vi "Save EPR Data-Rev3.vi"(5 "Save Data Type":T1, 7 "Spectral Data":T2={"PDT Amp [v]"=0.0, "RIS Amp [v]"=0.0, "B-Field"=[], "All In-Phase Scan Spectra"=[], "Model Select"=enum."OneCompRISTwoPDT", "Fit Each Scan"=FALSE, "PDT Center [g]"=0.0, "In-Phase Average Spectra"=[], "In-Phase Median Spectra"=[], "Out-Phase Median Spectra"=[], "Out-Phase Average Spectra"=[], "Fit Spectra"=[], "Fit No-Baseline Spectra"=[], "All Out-Phase Scan Spectra"=[], "Baseline Offset Correction"=FALSE, "In-Phase Offset [v]"=0.0, "Out-Phase Offset [v]"=0.0, "Ch2 Input\n(Balance)"=[], "Ch3 Input\n(Phase)"=[], "Ch4 Input\n(AFC)"=[], "Fit Pars"=[], "Fit Pars Errors"=[], "Fit Pars Labels"=[], "Raw Scan DAQ Data"=[], "Bad Scans Indicies"=[], "Good In-Phase Scan Spectra"=[], "Good Out-Phase Scan Spectra"=[], "Bad In-Phase Scan Spectra"=[], "Bad Out-Phase Scan Spectra"=[], "Number of bad scans"=0, "Fit History"=[], "PDT Amp. History/Set [v]"=[], "RIS Amp. History/Set [v]"=[], "RIS Amp. History/Scan [v]"=[], "All Shifted B-Fields"=[], "Good Shifted B-Fields"=[], "Ch5 Input\n(SpO2)"=[], "Ch6 Input\n(BPM)"=[], "Global SNR"=0.0, "Fit Error History"=[], "SNR History"=[]} {"Global SNR" min=0.0; "PDT Center [g]" min=0.0; "RIS Amp [v]" min=0.0; "PDT Amp [v]" min=0.0}, 8 "Measurement Information":T4={"Comments"="", "Directory Input"="", "Data file path"=path "C:/Data/EPR Data", "Scripting File"=path "C:/Data/Configuration Script.csv", "Save Data"=FALSE, "Tooth size (d11) [mm]"=0.0, "Tooth size (d12) [mm]"=0.0, "Tooth size (d21) [mm]"=0.0, "Tooth size (d22) [mm]"=0.0, "Dose of Tooth [Gy]"=0.0, "Safe Shutdown?"=FALSE, "Gases Available"=[], "Database Username"="", "Database Password"="", "Database Login URL"="", "Database Upload URL"="", "Database Success URL"="", "Database XML URL"="", "Database Resonator URL"="", "Session Number"=0, "Set #"=0, "Resonator Operator"="", "Session Type"="", "Tooth/Sample ID"="", "Volunteer ID"="", "Computer Operator"="", "Volunteer Type"="", "Site/Tooth Selection (T8,T9)"="", "Resonator"="", "Measurement Site"="", "Non-standard session?"=FALSE, "EPR DAQ Version"="", "Session Path"=path "C:/Data/EPR Data", "Chosen Applied State"="", "Chosen Initial State"="", "Time of Transition"="", "DAQ Mode"=enum."Engineering", "pO2/Scan [mmHg]"=[], "pO2/Set [mmHg]"=[], "Linewidth (HWHM)/Scan [Gauss]"=[], "Linewidth (HWHM)/Set [Gauss]"=[], "pO2 Conversion"="", "Dose Calibration Cluster"={"Dose Response"={"grand_mean"=0.0292016, "slope"=0.0188720543}, "Dose Correction"={"Sex"=1, "a0"=7.719669421, "a1"=-2.746550736, "a2"=-0.186490355, "a3"=0.041922063, "a4"=-0.849147359, "a5"=0.14330063, "a6"=0.019930219, "A_n"=40.0, "H_n"=10.12, "Dose Correction"=FALSE}, "Dose Reporting"={"Reporting is"=TRUE, "sd_threshold [AU]"=0.06, "sd_model [Gy]"=0.66, "dosimetric_threshold [Gy]"=2.0, "Add intrasession errors is"=FALSE, "Prior Radiation?"=FALSE}}, "OxyChip Slope"=0.0, "OxyChip Intercept"=0.0, "QA Mode"=enum."Select QA Mode", "QA Session?"=FALSE, "Sample Type"=enum."Empty Resonator", "Report pO2/Scan"=FALSE, "Skip End Session Save"=FALSE, "Number of sites"=enum."# Probes", "Recipient Name"="", "Sender Name"="", "Recipient Email"="", "Transition State History"=[], "pO2 Report Times"=[], "Temperature [C]"=0.0, "+Error pO2/Scan [mmHg]"=[], "-Error pO2/Scan [mmHg]"=[], "+Error pO2/Set [mmHg]"=[], "-Error pO2/Set [mmHg]"=[], "Oxy Phase Exclusion Tolerance [rad]"=0.0, "Oxy Center Exclusion Tolerance [%]"=0.0, "Oxy Exclude Unacceptable"=FALSE, "Oxy Unacceptable Estimate Flags"=[], "Save Session PPT"=FALSE, "Flagged Bad Sets"=[]} {"Oxy Center Exclusion Tolerance [%]" format="%#_9g"; "Oxy Phase Exclusion Tolerance [rad]" format="%#_9g"; "Temperature [C]" format="%#_9g"; "OxyChip Intercept" format="%#_9g"; "OxyChip Slope" format="%#_9g"; "Dose Calibration Cluster"."Dose Reporting"."dosimetric_threshold [Gy]" format="%#_9g"; "Dose Calibration Cluster"."Dose Reporting"."sd_model [Gy]" format="%#_9g"; "Dose Calibration Cluster"."Dose Reporting"."sd_threshold [AU]" format="%#_9g"; "Dose Calibration Cluster"."Dose Correction"."H_n" format="%#_9g"; "Dose Calibration Cluster"."Dose Correction"."A_n" format="%#_9g"; "Dose Calibration Cluster"."Dose Correction"."a6" format="%#.9g"; "Dose Calibration Cluster"."Dose Correction"."a5" format="%#.9g"; "Dose Calibration Cluster"."Dose Correction"."a4" format="%#.9g"; "Dose Calibration Cluster"."Dose Correction"."a3" format="%#.9g"; "Dose Calibration Cluster"."Dose Correction"."a2" format="%#.9g"; "Dose Calibration Cluster"."Dose Correction"."a1" format="%#.9g"; "Dose Calibration Cluster"."Dose Correction"."a0" format="%#.9g"; "Dose Calibration Cluster"."Dose Correction"."Sex" items=["Male"=1, "Female"=0]; "Dose Calibration Cluster"."Dose Response"."slope" format="%#_9g"; "Dose Calibration Cluster"."Dose Response"."grand_mean" format="%#_9g"}, 9 "Hardware Parameters":T7={"Scan Calibration [G/V]"=0.0, "Modulation Calibration [G/V]"=0.0, "Modulation Phase [deg]"=0.0, "Modulation Frequency [Hz]"=0.0, "Attenuation [dB]"=0, "Input Channel Count"=0, "Time constant"=7, "Sensitivity"=17, "Frequency Output Voltage [V]"=0.0, "Phase Output Voltage [V]"=0.0, "Lock-in Offset Compensation"=FALSE, "RF [GHz]"=0.0, "Q Start"=0.0, "Q End"=0.0, "Balance"=0.0, "Phase Error"=0.0, "AFC Error"=0.0, "AFC"=FALSE, "Magnet Rotation"=FALSE, "Balance Scaling Factor"=1.0, "Phase Error Scaling Factor"=1.0, "AFC Error Scaling Factor"=1.0, "Frequency Counter ID"="", "Sweep Waveform"=enum."Sawtooth", "Q-Factor Scale"=0.0, " Q-Data Scale"=0.0, " Q-Data Offset"=0.0, "Magnet Rotation Slope"=0.0, "Magnet Rotation Offset"=0.0, "Phase Sweep Resolution"=0.0, "Hardware Version Number"="", "Spectrometer ID Number"=0, "Spectrometer Name"="", "Lock in Saturation"=0.0, "Balance Threshold"=0.0, "Phase Error Threshold"=0.0, "AFC Error Threshold"=0.0, "Linear Actuator Length"=0.0, "Lock-in OK?"=FALSE, "Ignore Lock-in Comm. Failure"=FALSE, "Gradient Addresses"=[], "Gradient Calibrations [G/A*mm]"=[], "Gradient Power Supplies"=[], "Lock-in Address"="", "Magnet Type"=enum."RRI", "Camera Names"=[], "Sweep Limit [Gauss]"=0.0, "Modulation Limit [Gauss]"=0.0, "Balance Threshold Exceeded?"=FALSE, "Phase Threshold Exceeded?"=FALSE, "AFC Threshold Exceeded?"=FALSE, "Consecutive Re-tune attempts"=0, "Reverse Sweep Slope [sec]"=0.0, "Reverse Sweep Offset [G]"=0.0, "AFC Field Correction [V/MHz]"=0.0, "Active Gradients (X Y Z)"=[], "SpO2 Calibration [SpO2/V]"=1.0, "Heart Rate Calibration [BPM/V]"=1.0, "Thermocouple Channel"=""} {"Sensitivity" items=["", "2 nV", "5 nV", "10 nV", "20 nV", "50 nV", "100 nV", "200 nV", "500 nV", "1 uV", "2 uV", "5 uV", "10 uV", "20 uV", "50 uV", "100 uV", "200 uV", "500 uV", "1 mV", "2 mV", "5 mV", "10 mV", "20 mV", "50 mV", "100 mV", "200 mV", "500 mV", "1 V"]; "Time constant" items=["10 us", "20 us", "40 us", "80 us", "160 us", "320 us", "640 us", "5 ms", "10 ms", "20 ms", "50 ms", "100 ms", "200 ms", "500 ms", "1 s", "2 s", "5 s", "10 s", "20 s", "50 s", "100 s", "200 s", "500 s", "1 ks", "2 ks", "5 ks", "10 ks", "20 ks", "50 ks", "100 ks"]}, 10 "Acquisition Parameters":T8={"Magnet Angle [deg]"=0.0, "Magnet Angles [deg]"=[], "DeltaVpp [v]"=0.0, "SEM [v]"=0.0, "DeltaVpp Thresh [v]"=0.0, "SEM Thresh [v]"=0.0, "Adaptive Processing"=FALSE, "Acquire Q"=FALSE, "Acquire Photos"=FALSE, "Adaptive Tuning"=FALSE, "Automated Matching"=FALSE, "X-Gradient [G/mm]"=0.0, "Y-Gradient [G/mm]"=0.0, "Z-Gradient [G/mm]"=0.0, "Central Field [G]"=0.0, "Scan Width [G]"=0.0, "Mod. Amp. [G]"=0.0, "Scan Time [s]"=0.0, "Pre-Scan Delay [ms]"=0, "Measurement Timeout [s]"=0.0, "Electromagnet Main Field [G]"=0.0, "Locked Central Field [G]"=0.0, "Scans Excluded"=0, "Scans Completed"=0, "No. Scans/Set"=0, "No. Scans for SNR"=0, "Field Locked Frequency [GHz]"=0.0, "Auto Set-based Field Center"=FALSE, "Prompt for oxy acquisition updates"=FALSE, "Oxy QA Scan?"=FALSE, "Exclude Bad Data"=FALSE, "Optimizing RF Power"=FALSE, "Gradients on/off"=FALSE, "Running Script"=TRUE, "Opto-Coupler Current [A]"=0.0, "Continuous Sweeping"=FALSE, "Sweep Rise Time [sec]"=0, "Reverse Sweep Central Field [G]"=0.0, "Forward Sweep Central Field [G]"=0.0, "Sweep Calibrated"=FALSE, "Modulation Calibrated"=FALSE, "First CheckCal Scan?"=FALSE, "AFC Field Correction"=FALSE, "OxyQAInit Scan Width [G]"=0.0, "OxyQAInit Mod. Amp. [G]"=0.0, "Scans Completed/Session"=0, "Acquire SpO2"=FALSE, "Acquire Temperature"=FALSE, "Over Mod"=FALSE} {"OxyQAInit Mod. Amp. [G]" min=0.0; "OxyQAInit Scan Width [G]" min=0.0; "Mod. Amp. [G]" min=0.0; "Scan Width [G]" min=0.0; "Central Field [G]" min=0.0; "Measurement Timeout [s]" min=0.0; "Scan Time [s]" min=0.0; "Z-Gradient [G/mm]" min=0.0; "SEM Thresh [v]" min=0.0; "SEM [v]" min=0.0; "DeltaVpp [v]" min=0.0}) -> (3 "Filename":string)   [LabVIEW 2016]
uses:
  Types/Acquisition Parameters.ctl
  Types/Hardware Parameters.ctl
  Types/Measurement Information.ctl
  Analysis/Dose Calculation and Reporting/Dose Calculation Control.ctl
  Types/Sample Type.ctl
  Types/Spectral Data.ctl
  Types/Fitting Model Selection.ctl
  Types/Save Data Type.ctl
panel:
  # "Session Information"
  # "Oximetric Data and Information"
  # "Email"
  # "Tooth Information"
  # "Database"
  # "Bridge I/O"
  # "Magnet Rotation"
  # "Field Calibration"
  # "Lock In Amplifier"
  # "Spectrometer Information"
  # "DAQ Settings"
  # "Gradient Coils and Field"
  # "X"
  # "Y"
  # "Z"
  # "Q-Measurements"
  # "Gradients"
  # "Field"
  # "Scans and Sets"
  # "Timing"
  # "Adaptive Dosimetric \nData Processing"
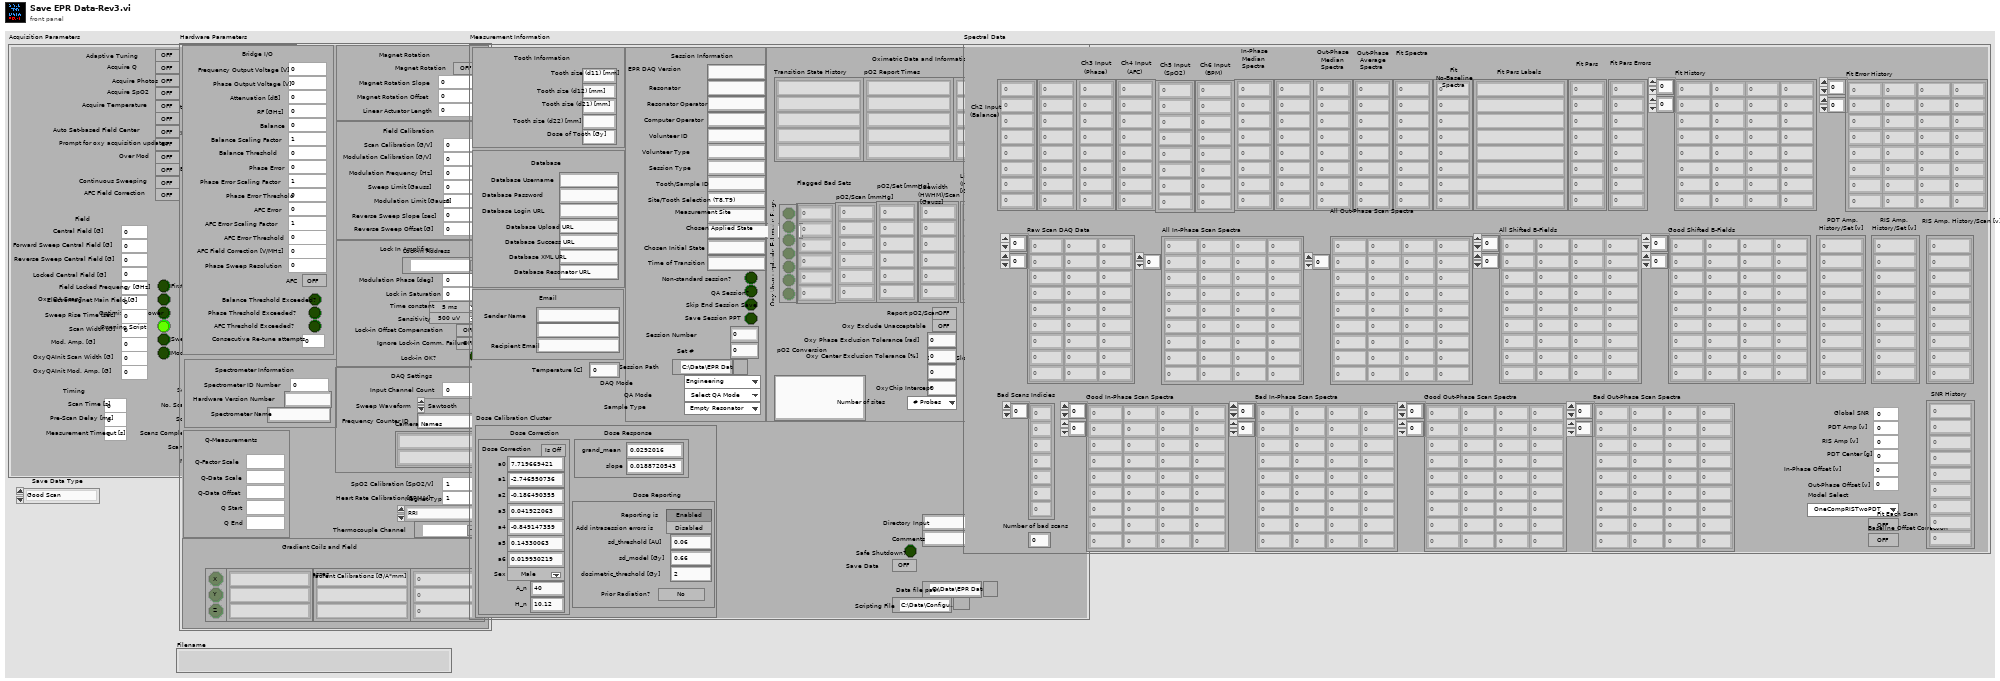
[diagram p1: front panel]
types:
  T1 = typedef "Save Data Type.ctl" = enum16{"Good Scan", "Bad Scan", "Appended Scans", "Median", "Filename"}
  T2 = typedef "Spectral Data.ctl" = cluster{"PDT Amp [v]":dbl, "RIS Amp [v]":dbl, "B-Field":dbl[], "All In-Phase Scan Spectra":dbl[][], "Model Select":T3, "Fit Each Scan":bool, "PDT Center [g]":dbl, "In-Phase Average Spectra":dbl[], "In-Phase Median Spectra":dbl[], "Out-Phase Median Spectra":dbl[], "Out-Phase Average Spectra":dbl[], "Fit Spectra":dbl[], "Fit No-Baseline Spectra":dbl[], "All Out-Phase Scan Spectra":dbl[][], "Baseline Offset Correction":bool, "In-Phase Offset [v]":dbl, "Out-Phase Offset [v]":dbl, "Ch2 Input\n(Balance)":dbl[], "Ch3 Input\n(Phase)":dbl[], "Ch4 Input\n(AFC)":dbl[], "Fit Pars":dbl[], "Fit Pars Errors":dbl[], "Fit Pars Labels":string[], "Raw Scan DAQ Data":dbl[][], "Bad Scans Indicies":i32[], "Good In-Phase Scan Spectra":dbl[][], "Good Out-Phase Scan Spectra":dbl[][], "Bad In-Phase Scan Spectra":dbl[][], "Bad Out-Phase Scan Spectra":dbl[][], "Number of bad scans":i32, "Fit History":dbl[][], "PDT Amp. History/Set [v]":dbl[], "RIS Amp. History/Set [v]":dbl[], "RIS Amp. History/Scan [v]":dbl[], "All Shifted B-Fields":dbl[][], "Good Shifted B-Fields":dbl[][], "Ch5 Input\n(SpO2)":dbl[], "Ch6 Input\n(BPM)":dbl[], "Global SNR":dbl, "Fit Error History":dbl[][], "SNR History":dbl[]}
  T3 = typedef "Fitting Model Selection.ctl" = enum16{"OneCompRIS", "OneCompRISTwoPDT", "OneCompRISRev", "OneCompRISTwoPDTRev", "LiPc", "TwoLiPc", "ThreeLiPc", "FourLiPc", "PDTCalibration", "CE_Ink", "Printex", "MelaninTwoPDT"}
  T4 = typedef "Measurement Information.ctl" = cluster{"Comments":string, "Directory Input":string, "Data file path":path, "Scripting File":path, "Save Data":bool, "Tooth size (d11) [mm]":dbl, "Tooth size (d12) [mm]":dbl, "Tooth size (d21) [mm]":dbl, "Tooth size (d22) [mm]":dbl, "Dose of Tooth [Gy]":dbl, "Safe Shutdown?":bool, "Gases Available":string[], "Database Username":string, "Database Password":string, "Database Login URL":string, "Database Upload URL":string, "Database Success URL":string, "Database XML URL":string, "Database Resonator URL":string, "Session Number":i32, "Set #":u32, "Resonator Operator":string, "Session Type":string, "Tooth/Sample ID":string, "Volunteer ID":string, "Computer Operator":string, "Volunteer Type":string, "Site/Tooth Selection (T8,T9)":string, "Resonator":string, "Measurement Site":string, "Non-standard session?":bool, "EPR DAQ Version":string, "Session Path":path, "Chosen Applied State":string, "Chosen Initial State":string, "Time of Transition":string, "DAQ Mode":enum16{"Engineering", "Dosimetry", "Oximetry"}, "pO2/Scan [mmHg]":dbl[][], "pO2/Set [mmHg]":dbl[][], "Linewidth (HWHM)/Scan [Gauss]":dbl[][], "Linewidth (HWHM)/Set [Gauss]":dbl[][], "pO2 Conversion":string, "Dose Calibration Cluster":T5, "OxyChip Slope":dbl, "OxyChip Intercept":dbl, "QA Mode":enum16{"Select QA Mode", "QA-Start/End", "QA-Mid", "QA-Weekly", "QA-Eng", "Check Calibration"}, "QA Session?":bool, "Sample Type":T6, "Report pO2/Scan":bool, "Skip End Session Save":bool, "Number of sites":enum16{"# Probes", "1", "2", "3", "4"}, "Recipient Name":string, "Sender Name":string, "Recipient Email":string, "Transition State History":string[], "pO2 Report Times":string[], "Temperature [C]":dbl, "+Error pO2/Scan [mmHg]":dbl[][], "-Error pO2/Scan [mmHg]":dbl[][], "+Error pO2/Set [mmHg]":dbl[][], "-Error pO2/Set [mmHg]":dbl[][], "Oxy Phase Exclusion Tolerance [rad]":dbl, "Oxy Center Exclusion Tolerance [%]":dbl, "Oxy Exclude Unacceptable":bool, "Oxy Unacceptable Estimate Flags":bool[], "Save Session PPT":bool, "Flagged Bad Sets":u32[]}
  T5 = typedef "Dose Calculation Control.ctl" = cluster{"Dose Response":cluster{"grand_mean":dbl, "slope":dbl}, "Dose Correction":cluster{"Sex":u16, "a0":dbl, "a1":dbl, "a2":dbl, "a3":dbl, "a4":dbl, "a5":dbl, "a6":dbl, "A_n":dbl, "H_n":dbl, "Dose Correction":bool}, "Dose Reporting":cluster{"Reporting is":bool, "sd_threshold [AU]":dbl, "sd_model [Gy]":dbl, "dosimetric_threshold [Gy]":dbl, "Add intrasession errors is":bool, "Prior Radiation?":bool}}
  T6 = typedef "Sample Type.ctl" = enum16{"Empty Resonator", "IRS", "BallZero", "Irradiated Tooth", "Non-irradiated Tooth", "OxyChip", "LiPc", "PDT", "India Ink"}
  T7 = typedef "Hardware Parameters.ctl" = cluster{"Scan Calibration [G/V]":dbl, "Modulation Calibration [G/V]":dbl, "Modulation Phase [deg]":dbl, "Modulation Frequency [Hz]":dbl, "Attenuation [dB]":u16, "Input Channel Count":i32, "Time constant":u16, "Sensitivity":u16, "Frequency Output Voltage [V]":dbl, "Phase Output Voltage [V]":dbl, "Lock-in Offset Compensation":bool, "RF [GHz]":dbl, "Q Start":dbl, "Q End":dbl, "Balance":dbl, "Phase Error":dbl, "AFC Error":dbl, "AFC":bool, "Magnet Rotation":bool, "Balance Scaling Factor":dbl, "Phase Error Scaling Factor":dbl, "AFC Error Scaling Factor":dbl, "Frequency Counter ID":string, "Sweep Waveform":enum16{"Sine Wave", "Square Wave", "Sawtooth", "Triangle Wave"}, "Q-Factor Scale":dbl, " Q-Data Scale":dbl, " Q-Data Offset":dbl, "Magnet Rotation Slope":dbl, "Magnet Rotation Offset":dbl, "Phase Sweep Resolution":dbl, "Hardware Version Number":string, "Spectrometer ID Number":i32, "Spectrometer Name":string, "Lock in Saturation":dbl, "Balance Threshold":dbl, "Phase Error Threshold":dbl, "AFC Error Threshold":dbl, "Linear Actuator Length":dbl, "Lock-in OK?":bool, "Ignore Lock-in Comm. Failure":bool, "Gradient Addresses":string[], "Gradient Calibrations [G/A*mm]":dbl[], "Gradient Power Supplies":string[], "Lock-in Address":refnum<visa-resource-name>, "Magnet Type":enum16{"RRI", "BARDA", "Whole Body Permanent", "RRI Electromagnet"}, "Camera Names":string[], "Sweep Limit [Gauss]":dbl, "Modulation Limit [Gauss]":dbl, "Balance Threshold Exceeded?":bool, "Phase Threshold Exceeded?":bool, "AFC Threshold Exceeded?":bool, "Consecutive Re-tune attempts":i32, "Reverse Sweep Slope [sec]":dbl, "Reverse Sweep Offset [G]":dbl, "AFC Field Correction [V/MHz]":dbl, "Active Gradients (X Y Z)":bool[], "SpO2 Calibration [SpO2/V]":dbl, "Heart Rate Calibration [BPM/V]":dbl, "Thermocouple Channel":tag}
  T8 = typedef "Acquisition Parameters.ctl" = cluster{"Magnet Angle [deg]":dbl, "Magnet Angles [deg]":dbl[], "DeltaVpp [v]":dbl, "SEM [v]":dbl, "DeltaVpp Thresh [v]":dbl, "SEM Thresh [v]":dbl, "Adaptive Processing":bool, "Acquire Q":bool, "Acquire Photos":bool, "Adaptive Tuning":bool, "Automated Matching":bool, "X-Gradient [G/mm]":dbl, "Y-Gradient [G/mm]":dbl, "Z-Gradient [G/mm]":dbl, "Central Field [G]":dbl, "Scan Width [G]":dbl, "Mod. Amp. [G]":dbl, "Scan Time [s]":dbl, "Pre-Scan Delay [ms]":u32, "Measurement Timeout [s]":dbl, "Electromagnet Main Field [G]":dbl, "Locked Central Field [G]":dbl, "Scans Excluded":u32, "Scans Completed":u32, "No. Scans/Set":u32, "No. Scans for SNR":u32, "Field Locked Frequency [GHz]":dbl, "Auto Set-based Field Center":bool, "Prompt for oxy acquisition updates":bool, "Oxy QA Scan?":bool, "Exclude Bad Data":bool, "Optimizing RF Power":bool, "Gradients on/off":bool, "Running Script":bool, "Opto-Coupler Current [A]":dbl, "Continuous Sweeping":bool, "Sweep Rise Time [sec]":u32, "Reverse Sweep Central Field [G]":dbl, "Forward Sweep Central Field [G]":dbl, "Sweep Calibrated":bool, "Modulation Calibrated":bool, "First CheckCal Scan?":bool, "AFC Field Correction":bool, "OxyQAInit Scan Width [G]":dbl, "OxyQAInit Mod. Amp. [G]":dbl, "Scans Completed/Session":u32, "Acquire SpO2":bool, "Acquire Temperature":bool, "Over Mod":bool}
  T9 = enum16{"RRI", "BARDA", "Whole Body Permanent", "RRI Electromagnet"}
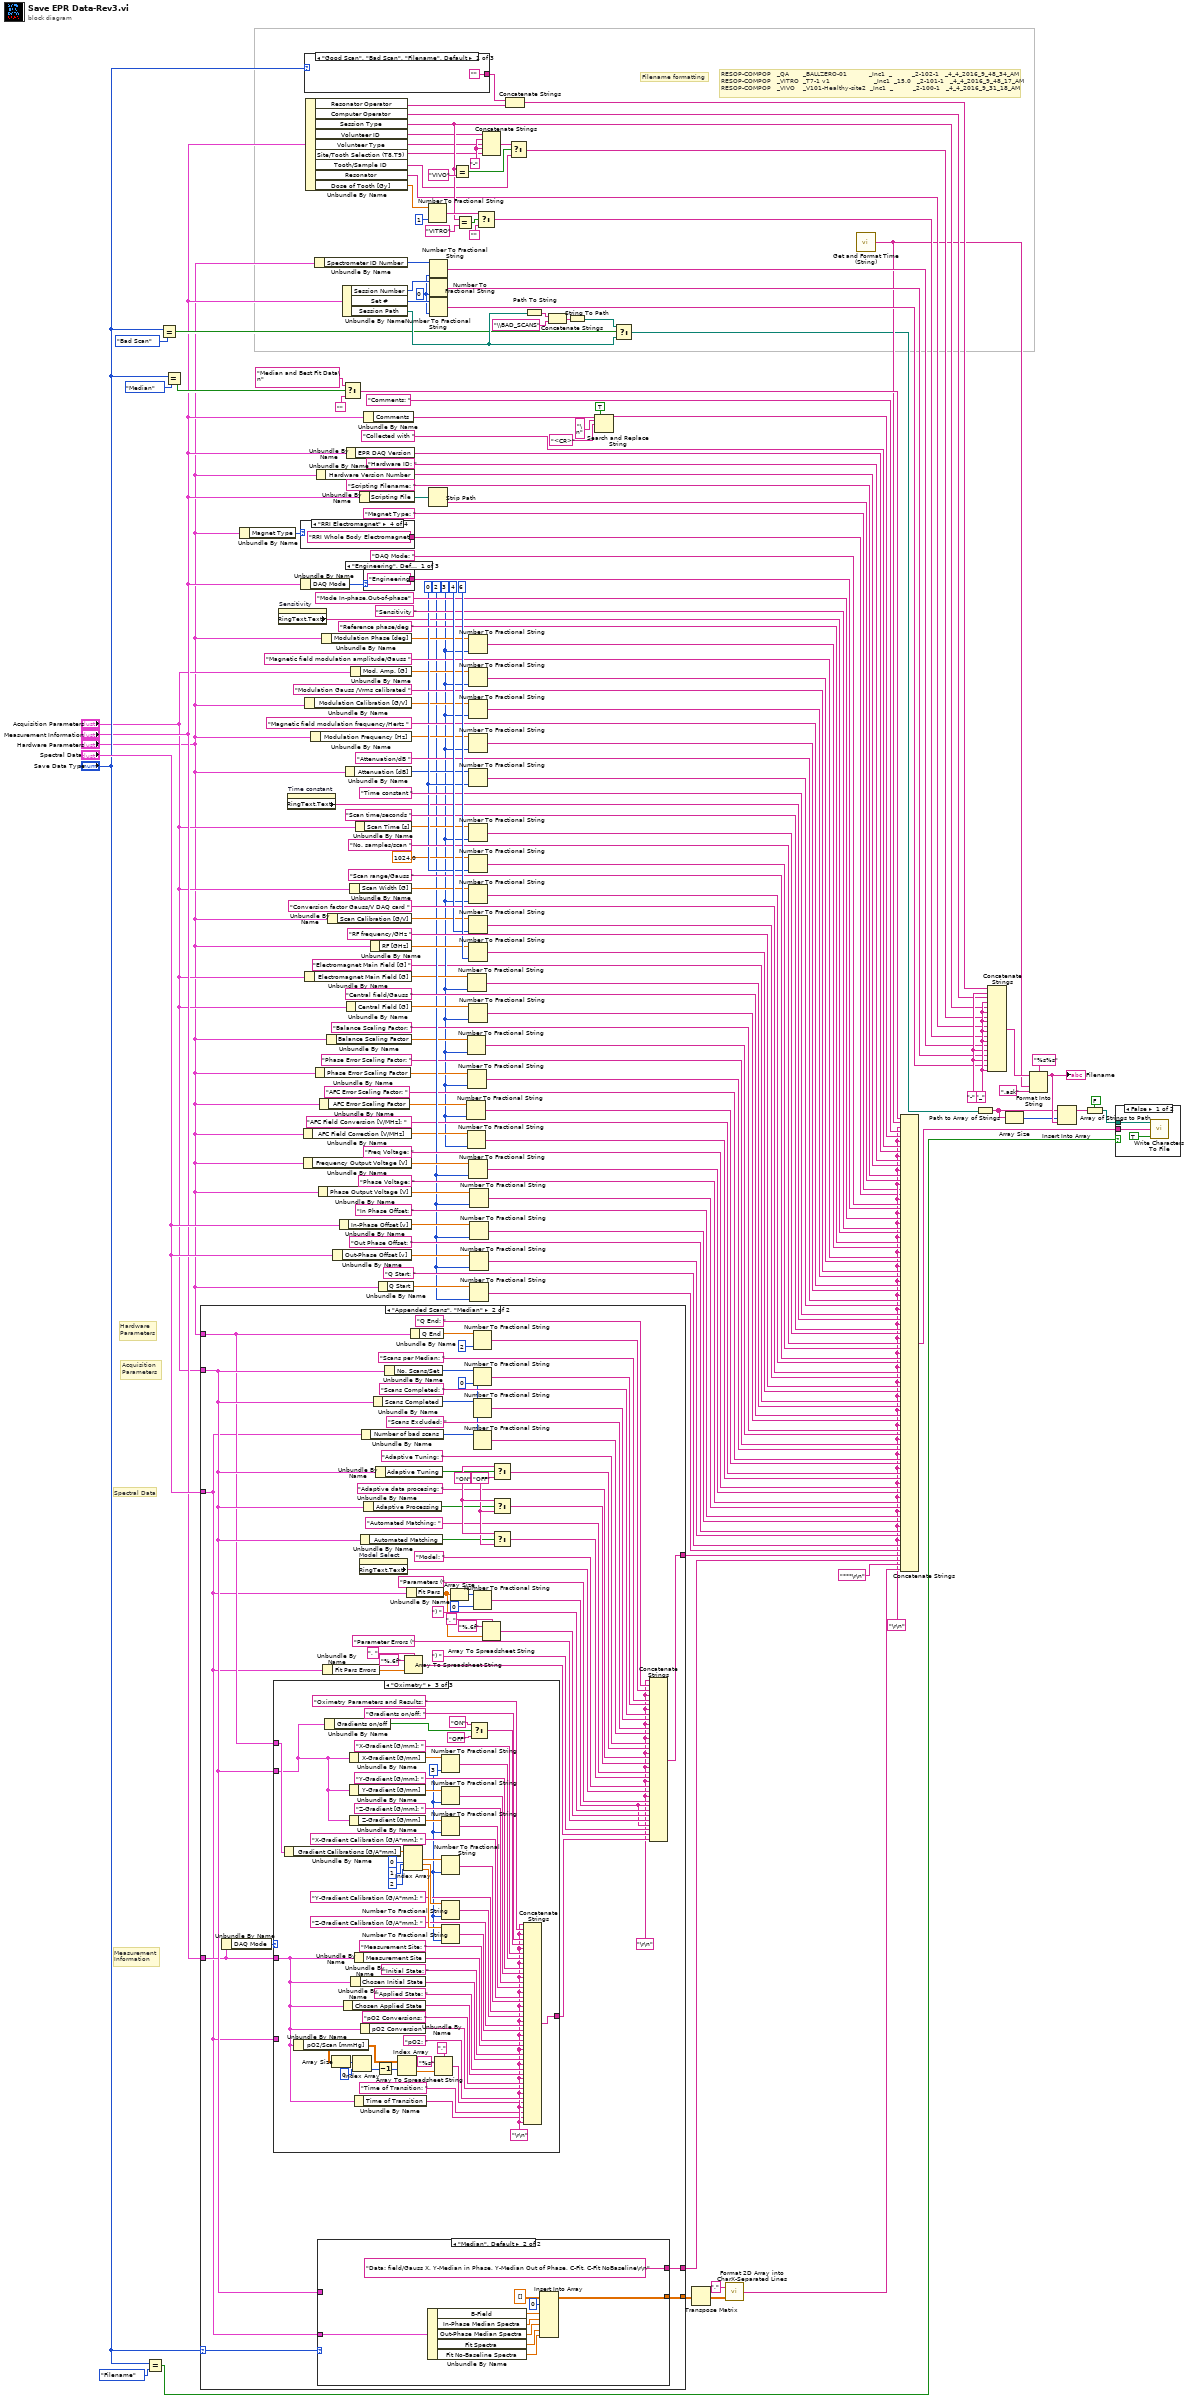
[diagram p0: block diagram]
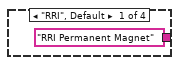
[diagram p2: hidden frame]
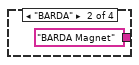
[diagram p3: hidden frame]
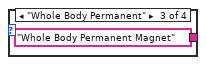
[diagram p4: hidden frame]
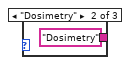
[diagram p5: hidden frame]
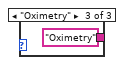
[diagram p6: hidden frame]
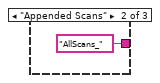
[diagram p7: hidden frame]
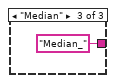
[diagram p8: hidden frame]
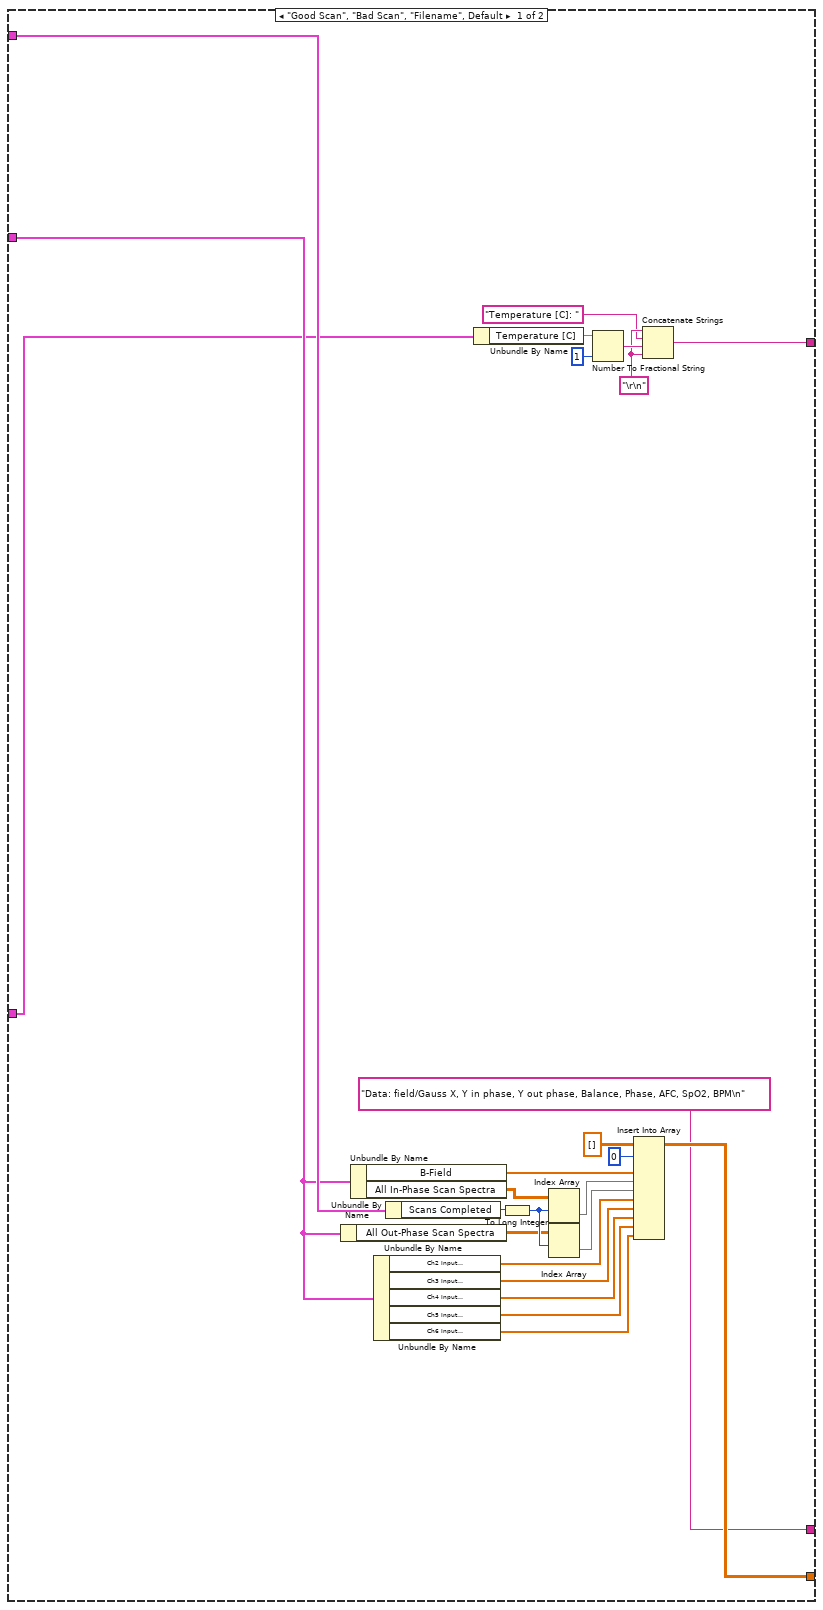
[diagram p10: hidden frame]
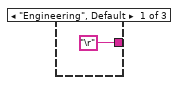
[diagram p11: hidden frame]
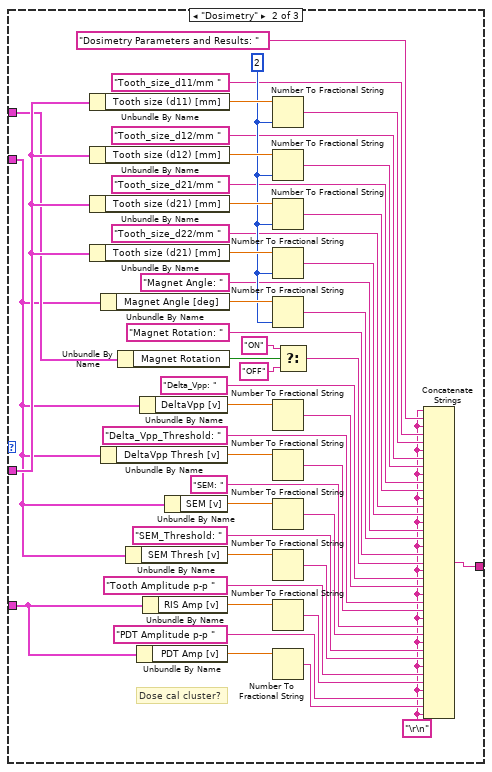
[diagram p12: hidden frame]
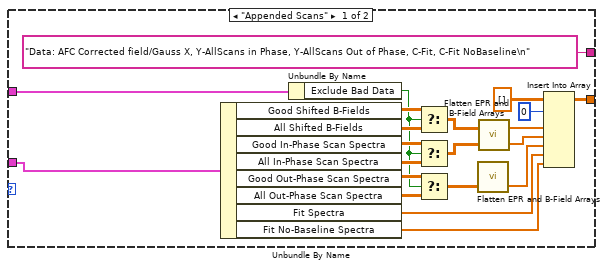
[diagram p13: hidden frame]
diagram:
  w49 = i16 0 ("width (-)")
  w100 = "-" ("string")
  w108 = i16 0 ("precision (6)")
  w8 = i16 3 ("precision (6)")
  w104 = "-" ("string")
  w3 = "\r\n" ("string")
  w33 = i16 2 ("precision (6)")
  w105 = "_" ("string")
  # "Measurement\nInformation"
  # "Spectral Data"
  # "Hardware \nParameters"
  # "Acquisition \nParameters"
  # "Filename formatting"
  # "RESOP-COMPOP   _QA       _BALLZERO-01           _Inc1  _          _2-102-1   _4_4_2016_9_48_34_AM\nRESOP-COMPOP   _VITRO  _T7-1 v1                      _Inc1  _15.0   _2-101-1   _4_4_2016_9_48_17_AM\nRESOP-COMPOP   _VIVO    _V101-Healthy-site2  _Inc1  _          _2-100-1   _4_4_2016_9_31_18_AM"
  n1 = Equal?(x="Save Data Type", y=Save_Data_Type."Filename" ("Save Data Type")) -> (x = y?=w35:bool)
  n2 = Equal?(x="Save Data Type", y=Save_Data_Type."Bad Scan" ("Save Data Type")) -> (x = y?=w37:bool)
  n3 = Equal?(x="Save Data Type", y=Save_Data_Type."Median" ("Save Data Type")) -> (x = y?=w39:bool)
  n4 = case shown="\"Appended Scans\", \"Median\"" "Save Data Type" {
    selector: "Save Data Type" -> [_ w207]
    tunnel: [w165 w238] -> w107
    tunnel: "Hardware Parameters" -> [_ w192]
    tunnel: "Acquisition Parameters" -> [w175 w193]
    tunnel: "Spectral Data" -> [w174 w188]
    tunnel: [w176 w219] -> w66
    tunnel: ["Data: field/Gauss X, Y in phase, Y out phase, Balance, Phase, AFC, SpO2, BPM\n" ("string") w206] -> w65
    tunnel: "Measurement Information" -> [w169 w190]
    frame "Good Scan", "Bad Scan", "Filename", Default {
      w164 = "\r\n" ("string")
      n5 = Unbundle By Name(w174) -> ("All Out-Phase Scan Spectra"=w178:dbl[][])
      n6 = Unbundle By Name(w174) -> ("B-Field"=w184:dbl[], "All In-Phase Scan Spectra"=w172:dbl[][])
      n7 = Unbundle By Name(w174) -> ("Ch2 Input\n(Balance)"=w181:dbl[], "Ch3 Input\n(Phase)"=w182:dbl[], "Ch4 Input\n(AFC)"=w183:dbl[], "Ch5 Input\n(SpO2)"=w171:dbl[], "Ch6 Input\n(BPM)"=w170:dbl[])
      n8 = Unbundle By Name(w175) -> ("Scans Completed"=w177:u32)
      n9 = Unbundle By Name(w169) -> ("Temperature [C]"=w168:dbl)
      n10 = To Long Integer(number=w177) -> (32bit integer=w179:i32)
      n11 = Index Array(array=w172, index (row)=w179) -> (element=w185:dbl[])  [unwired: 1 in]
      n12 = Index Array(array=w178, index (row)=w179) -> (element=w180:dbl[])  [unwired: 1 in]
      n13 = Number To Fractional String(number=w168, precision (6)=i16 1) -> (F-format string=w166:string)  [unwired: 2 in]
      n14 = Insert Into Array(array=dbl[][] [] ("In-Phase Scan Spectras"), index (row)=0, new element #1=w184, new element #2=w185, new element #3=w180, new element #4=w181, new element #5=w182, new element #6=w183, new element #7=w171, new element #8=w170) -> (w176:dbl[][])  [unwired: 1 in]
      n15 = Concatenate Strings(w164, "Temperature [C]: " ("string"), w166, w164) -> (w165:string)
    }
    frame "Appended Scans", "Median" {
      w204 = "OFF" ("string")
      w205 = "ON" ("string")
      w226 = i16 0 ("precision (6)")
      w189 = "\r\n" ("string")
      n16 = Unbundle By Name(w190) -> ("DAQ Mode"=w194:enum16{"Engineering", "Dosimetry", "Oximetry"})
      n17 = case shown="\"Oximetry\"" w194 {
        tunnel: ["\r" w248 w341] -> w191
        tunnel: w193 -> [_ w243 w289]
        tunnel: w192 -> [_ w244 w325]
        tunnel: w190 -> [_ w245 w299]
        tunnel: w188 -> [_ w242 _]
        frame "Engineering", Default {
        }
        frame "Dosimetry" {
          w246 = "\r\n" ("string")
          w282 = i16 2 ("precision (6)")
          # "Dose cal cluster?"
          n18 = Unbundle By Name(w245) -> ("Tooth size (d11) [mm]"=w287:dbl)
          n19 = Unbundle By Name(w245) -> ("Tooth size (d12) [mm]"=w284:dbl)
          n20 = Unbundle By Name(w245) -> ("Tooth size (d21) [mm]"=w285:dbl)
          n21 = Unbundle By Name(w245) -> ("Tooth size (d21) [mm]"=w286:dbl)
          n22 = Unbundle By Name(w243) -> ("Magnet Angle [deg]"=w283:dbl)
          n23 = Unbundle By Name(w243) -> ("DeltaVpp Thresh [v]"=w278:dbl)
          n24 = Unbundle By Name(w244) -> ("Magnet Rotation"=w281:bool)
          n25 = Unbundle By Name(w243) -> ("SEM Thresh [v]"=w263:dbl)
          n26 = Unbundle By Name(w242) -> ("PDT Amp [v]"=w261:dbl)
          n27 = Unbundle By Name(w243) -> ("DeltaVpp [v]"=w265:dbl)
          n28 = Unbundle By Name(w242) -> ("RIS Amp [v]"=w262:dbl)
          n29 = Unbundle By Name(w243) -> ("SEM [v]"=w264:dbl)
          n30 = Number To Fractional String(number=w287, precision (6)=w282) -> (F-format string=w276:string)  [unwired: 2 in]
          n31 = Number To Fractional String(number=w284, precision (6)=w282) -> (F-format string=w274:string)  [unwired: 2 in]
          n32 = Number To Fractional String(number=w285, precision (6)=w282) -> (F-format string=w272:string)  [unwired: 2 in]
          n33 = Number To Fractional String(number=w286, precision (6)=w282) -> (F-format string=w270:string)  [unwired: 2 in]
          n34 = Number To Fractional String(number=w283, precision (6)=w282) -> (F-format string=w268:string)  [unwired: 2 in]
          n35 = Number To Fractional String(number=w265) -> (F-format string=w259:string)  [unwired: 3 in]
          n36 = Number To Fractional String(number=w278) -> (F-format string=w257:string)  [unwired: 3 in]
          n37 = Number To Fractional String(number=w264) -> (F-format string=w255:string)  [unwired: 3 in]
          n38 = Number To Fractional String(number=w263) -> (F-format string=w253:string)  [unwired: 3 in]
          n39 = Number To Fractional String(number=w262) -> (F-format string=w251:string)  [unwired: 3 in]
          n40 = Number To Fractional String(number=w261) -> (F-format string=w249:string)  [unwired: 3 in]
          n41 = Select(t="ON" ("string"), s=w281, f="OFF" ("string")) -> (s? t:f=w266:string)
          n42 = Concatenate Strings(w246, "Dosimetry Parameters and Results: " ("string"), w246, "Tooth_size_d11/mm " ("string"), w276, w246, "Tooth_size_d12/mm " ("string"), w274, w246, "Tooth_size_d21/mm " ("string"), w272, w246, "Tooth_size_d22/mm " ("string"), w270, w246, "Magnet Angle: " ("string"), w268, w246, "Magnet Rotation: " ("string"), w266, w246, "Delta_Vpp: " ("string"), w259, w246, "Delta_Vpp_Threshold: " ("string"), w257, w246, "SEM: " ("string"), w255, w246, "SEM_Threshold: " ("string"), w253, w246, "Tooth Amplitude p-p " ("string"), w251, w246, "PDT Amplitude p-p " ("string"), w249, w246) -> (w248:string)
        }
        frame "Oximetry" {
          w303 = i16 3 ("precision (6)")
          w302 = "\r\n" ("string")
          n43 = Unbundle By Name(w325) -> ("Gradient Calibrations [G/A*mm]"=w324:dbl[])
          n44 = Unbundle By Name(w299) -> ("pO2/Scan [mmHg]"=w296:dbl[][])
          n45 = Unbundle By Name(w289) -> ("Gradients on/off"=w288:bool)
          n46 = Array Size(array=w296) -> (size(s)=w298:i32[])
          n47 = Unbundle By Name(w299) -> ("Chosen Applied State"=w307:string)
          n48 = Unbundle By Name(w289) -> ("X-Gradient [G/mm]"=w334:dbl)
          n49 = Unbundle By Name(w289) -> ("Y-Gradient [G/mm]"=w333:dbl)
          n50 = Unbundle By Name(w289) -> ("Z-Gradient [G/mm]"=w328:dbl)
          n51 = Unbundle By Name(w299) -> ("Chosen Initial State"=w309:string)
          n52 = Index Array(array=w298, index=0) -> (element=w291:i32)
          n53 = Unbundle By Name(w299) -> ("Measurement Site"=w311:string)
          n54 = Unbundle By Name(w299) -> ("Time of Transition"=w300:string)
          n55 = Unbundle By Name(w299) -> ("pO2 Conversion"=w305:string)
          n56 = Decrement(x=w291) -> (x-1=w290:i32)
          n57 = Index Array(array=w296, index (row)=w290) -> (element=w293:dbl[])  [unwired: 1 in]
          n58 = Index Array(array=w324, index #1=0 ("index"), index #2=1 ("index"), index #3=2 ("index")) -> (element #1=w320:dbl, element #2=w319:dbl, element #3=w318:dbl)
          n59 = Array To Spreadsheet String(delimiter (Tab)=",", array=w293, 3:"%s" ("format string")) -> (spreadsheet string=w292:string)
          n60 = Number To Fractional String(number=w334, precision (6)=w303) -> (F-format string=w332:string)  [unwired: 2 in]
          n61 = Number To Fractional String(number=w333, precision (6)=w303) -> (F-format string=w330:string)  [unwired: 2 in]
          n62 = Number To Fractional String(number=w328, precision (6)=w303) -> (F-format string=w327:string)  [unwired: 2 in]
          n63 = Number To Fractional String(number=w320, precision (6)=w303) -> (F-format string=w317:string)  [unwired: 2 in]
          n64 = Number To Fractional String(number=w319, precision (6)=w303) -> (F-format string=w315:string)  [unwired: 2 in]
          n65 = Number To Fractional String(number=w318, precision (6)=w303) -> (F-format string=w313:string)  [unwired: 2 in]
          n66 = Select(t="ON" ("string"), s=w288, f="OFF" ("string")) -> (s? t:f=w335:string)
          n67 = Concatenate Strings(w302, "Oximetry Parameters and Results: " ("string"), w302, "Gradients on/off: " ("string"), w335, w302, "X-Gradient [G/mm]: " ("string"), w332, w302, "Y-Gradient [G/mm]: " ("string"), w330, w302, "Z-Gradient [G/mm]: " ("string"), w327, w302, "X-Gradient Calibration [G/A*mm]: " ("string"), w317, w302, "Y-Gradient Calibration [G/A*mm]: " ("string"), w315, w302, "Z-Gradient Calibration [G/A*mm]: " ("string"), w313, w302, "Measurement Site: " ("string"), w311, w302, "Initial State: " ("string"), w309, w302, "Applied State: " ("string"), w307, w302, "pO2 Conversions: " ("string"), w305, w302, "pO2: " ("string"), w292, w302, "Time of Transition: " ("string"), w300, w302) -> (w341:string)
        }
      }
      n68 = case shown="\"Median\", Default" w207 {
        tunnel: [w344 w369] -> w219
        tunnel: w188 -> [w343 w364]
        tunnel: ["Data: AFC Corrected field/Gauss X, Y-AllScans in Phase, Y-AllScans Out of Phase, C-Fit, C-Fit NoBaseline\n" ("string") "Data: field/Gauss X, Y-Median in Phase, Y-Median Out of Phase, C-Fit, C-Fit NoBaseline\r\n" ("string")] -> w206
        tunnel: w193 -> [w342 _]
        frame "Appended Scans" {
          n69 = Unbundle By Name(w343) -> ("Good Shifted B-Fields"=w360:dbl[][], "All Shifted B-Fields"=w359:dbl[][], "Good In-Phase Scan Spectra"=w358:dbl[][], "All In-Phase Scan Spectra"=w357:dbl[][], "Good Out-Phase Scan Spectra"=w356:dbl[][], "All Out-Phase Scan Spectra"=w355:dbl[][], "Fit Spectra"=w347:dbl[], "Fit No-Baseline Spectra"=w346:dbl[])
          n70 = Unbundle By Name(w342) -> ("Exclude Bad Data"=w348:bool)
          n71 = Select(t=w360, s=w348, f=w359) -> (s? t:f=w353:dbl[][])
          n72 = Select(t=w358, s=w348, f=w357) -> (s? t:f=w354:dbl[][])
          n73 = Select(t=w356, s=w348, f=w355) -> (s? t:f=w352:dbl[][])
          n74 = call "Flatten EPR and B-Field Arrays.vi"("2D EPR Data"=w352) -> ("1D Flattened EPR Data"=w349:dbl[])  [unwired: 1 in, 1 out]
          n75 = call "Flatten EPR and B-Field Arrays.vi"("2D EPR Data"=w354, "2D B-Fields"=w353) -> ("1D Flattened EPR Data"=w350:dbl[], "1D Flattened B-Fields"=w351:dbl[])
          n76 = Insert Into Array(array=dbl[][] [] ("In-Phase Scan Spectras"), index (row)=0, new element #1=w351, new element #2=w350, new element #3=w349, new element #4=w347, new element #5=w346) -> (w344:dbl[][])  [unwired: 1 in]
        }
        frame "Median", Default {
          n77 = Unbundle By Name(w364) -> ("B-Field"=w370:dbl[], "In-Phase Median Spectra"=w368:dbl[], "Out-Phase Median Spectra"=w367:dbl[], "Fit Spectra"=w366:dbl[], "Fit No-Baseline Spectra"=w365:dbl[])
          n78 = Insert Into Array(array=dbl[][] [] ("In-Phase Scan Spectras"), index (row)=0, new element #1=w370, new element #2=w368, new element #3=w367, new element #4=w366, new element #5=w365) -> (w369:dbl[][])  [unwired: 1 in]
        }
      }
      n79 = Unbundle By Name(w188) -> ("Fit Pars Errors"=w217:dbl[])
      n80 = property on="Model Select" class="Enum (strict)"() -> ("RingText.Text"=w218:string)  [unwired: 2 in, 2 out]
      n81 = Unbundle By Name(w193) -> ("Automated Matching"=w203:bool)
      n82 = Unbundle By Name(w188) -> ("Number of bad scans"=w221:i32)
      n83 = Unbundle By Name(w193) -> ("Adaptive Processing"=w202:bool)
      n84 = Unbundle By Name(w193) -> ("Scans Completed"=w222:u32)
      n85 = Unbundle By Name(w193) -> ("Adaptive Tuning"=w201:bool)
      n86 = Unbundle By Name(w193) -> ("No. Scans/Set"=w223:u32)
      n87 = Array To Spreadsheet String(delimiter (Tab)=", ", array=w217, 3:"%.6f" ("format string")) -> (spreadsheet string=w215:string)
      n88 = Unbundle By Name(w188) -> ("Fit Pars"=w211:dbl[])
      n89 = Unbundle By Name(w192) -> ("Q End"=w224:dbl)
      n90 = Array Size(array=w211) -> (size(s)=w220:i32)
      n91 = Number To Fractional String(number=w224, precision (6)=i16 2) -> (F-format string=w239:string)  [unwired: 2 in]
      n92 = Number To Fractional String(number=w223, precision (6)=w226) -> (F-format string=w236:string)  [unwired: 2 in]
      n93 = Number To Fractional String(number=w222, precision (6)=w226) -> (F-format string=w234:string)  [unwired: 2 in]
      n94 = Number To Fractional String(number=w221, precision (6)=w226) -> (F-format string=w232:string)  [unwired: 2 in]
      n95 = Number To Fractional String(number=w220, precision (6)=i16 0) -> (F-format string=w209:string)  [unwired: 2 in]
      n96 = Array To Spreadsheet String(delimiter (Tab)=", ", array=w211, 3:"%.6f" ("format string")) -> (spreadsheet string=w210:string)
      n97 = Select(t=w205, s=w201, f=w204) -> (s? t:f=w199:string)
      n98 = Select(t=w205, s=w202, f=w204) -> (s? t:f=w197:string)
      n99 = Select(t=w205, s=w203, f=w204) -> (s? t:f=w195:string)
      n100 = Concatenate Strings(w189, "Q End: " ("string"), w239, w189, "Scans per Median: " ("string"), w236, w189, "Scans Completed: " ("string"), w234, w189, "Scans Excluded: " ("string"), w232, w189, "Adaptive Tuning: " ("string"), w199, w189, "Adaptive data procesing: " ("string"), w197, w189, "Automated Matching: " ("string"), w195, w189, "Model: " ("string"), w218, w189, "Parameters (" ("string"), w209, ") " ("string"), w210, "Parameter Errors (" ("string"), w209, ") " ("string"), w215, w191) -> (w238:string)
    }
  }
  n101 = Unbundle By Name("Hardware Parameters") -> ("Magnet Type"=w5:T9)
  n102 = property on="Sensitivity" class="Ring (strict)"() -> ("RingText.Text"=w86:string)  [unwired: 2 in, 2 out]
  n103 = property on="Time constant" class="Ring (strict)"() -> ("RingText.Text"=w87:string)  [unwired: 2 in, 2 out]
  n104 = case shown="\"RRI Electromagnet\"" w5 {
    tunnel: ["RRI Permanent Magnet" ("string") "BARDA Magnet" ("string") "Whole Body Permanent Magnet" ("string") "RRI Whole Body Electromagnet" ("string")] -> w1
    frame "RRI", Default {
    }
    frame "BARDA" {
    }
    frame "Whole Body Permanent" {
    }
    frame "RRI Electromagnet" {
    }
  }
  n105 = Unbundle By Name("Measurement Information") -> ("DAQ Mode"=w22:enum16{"Engineering", "Dosimetry", "Oximetry"})
  n106 = Unbundle By Name("Hardware Parameters") -> ("AFC Field Correction [V/MHz]"=w21:dbl)
  n107 = Unbundle By Name("Hardware Parameters") -> ("Frequency Output Voltage [V]"=w73:dbl)
  n108 = case shown="\"Good Scan\", \"Bad Scan\", \"Filename\", Default" "Save Data Type" {
    tunnel: ["" "AllScans_" ("string") "Median_" ("string")] -> w41
    frame "Good Scan", "Bad Scan", "Filename", Default {
    }
    frame "Appended Scans" {
    }
    frame "Median" {
    }
  }
  n109 = Unbundle By Name("Hardware Parameters") -> ("Modulation Calibration [G/V]"=w83:dbl)
  n110 = Unbundle By Name("Acquisition Parameters") -> ("Electromagnet Main Field [G]"=w9:dbl)
  n111 = Unbundle By Name("Measurement Information") -> ("Resonator Operator"=w64:string, "Computer Operator"=w63:string, "Session Type"=w62:string, "Volunteer ID"=w61:string, "Volunteer Type"=w60:string, "Site/Tooth Selection (T8,T9)"=w59:string, "Tooth/Sample ID"=w58:string, "Resonator"=w57:string, "Dose of Tooth [Gy]"=w56:dbl)
  n112 = Unbundle By Name("Hardware Parameters") -> ("Modulation Frequency [Hz]"=w82:dbl)
  n113 = Unbundle By Name("Hardware Parameters") -> ("Spectrometer ID Number"=w55:i32)
  n114 = Unbundle By Name("Hardware Parameters") -> ("Phase Error Scaling Factor"=w28:dbl)
  n115 = Unbundle By Name("Hardware Parameters") -> ("Hardware Version Number"=w15:string)
  n116 = Unbundle By Name("Hardware Parameters") -> ("Phase Output Voltage [V]"=w72:dbl)
  n117 = Unbundle By Name("Hardware Parameters") -> ("AFC Error Scaling Factor"=w25:dbl)
  n118 = Unbundle By Name("Hardware Parameters") -> ("Modulation Phase [deg]"=w85:dbl)
  n119 = Unbundle By Name("Hardware Parameters") -> ("Balance Scaling Factor"=w31:dbl)
  n120 = Unbundle By Name("Hardware Parameters") -> ("Scan Calibration [G/V]"=w77:dbl)
  n121 = Unbundle By Name("Spectral Data") -> ("Out-Phase Offset [v]"=w70:dbl)
  n122 = Unbundle By Name("Spectral Data") -> ("In-Phase Offset [v]"=w71:dbl)
  n123 = Unbundle By Name("Measurement Information") -> ("Session Number"=w53:i32, "Set #"=w52:u32, "Session Path"=w44:path)
  n124 = Select(t="Median and Best Fit Data\n" ("string"), s=w39, f="") -> (s? t:f=w91:string)
  n125 = Unbundle By Name("Hardware Parameters") -> ("Attenuation [dB]"=w81:u16)
  n126 = Unbundle By Name("Measurement Information") -> ("EPR DAQ Version"=w17:string)
  n127 = Unbundle By Name("Acquisition Parameters") -> ("Central Field [G]"=w75:dbl)
  n128 = Unbundle By Name("Acquisition Parameters") -> ("Scan Width [G]"=w78:dbl)
  n129 = Unbundle By Name("Acquisition Parameters") -> ("Mod. Amp. [G]"=w84:dbl)
  n130 = Unbundle By Name("Acquisition Parameters") -> ("Scan Time [s]"=w80:dbl)
  n131 = Unbundle By Name("Measurement Information") -> ("Scripting File"=w74:path)
  n132 = case shown="\"Engineering\", Default" w22 {
    tunnel: ["Engineering" ("string") "Dosimetry" ("string") "Oximetry" ("string")] -> w11
    frame "Engineering", Default {
    }
    frame "Dosimetry" {
    }
    frame "Oximetry" {
    }
  }
  n133 = Unbundle By Name("Measurement Information") -> ("Comments"=w88:string)
  n134 = Unbundle By Name("Hardware Parameters") -> ("RF [GHz]"=w76:dbl)
  n135 = Unbundle By Name("Hardware Parameters") -> ("Q Start"=w69:dbl)
  n136 = Number To Fractional String(number=w56, precision (6)=i16 1) -> (F-format string=w95:string)  [unwired: 2 in]
  n137 = Strip Path(path=w74) -> (name=w13:string)  [unwired: 1 out]
  n138 = Number To Fractional String(number=w55, precision (6)=w49) -> (F-format string=w54:string)  [unwired: 2 in]
  n139 = Number To Fractional String(number=w53, precision (6)=w49) -> (F-format string=w51:string)  [unwired: 2 in]
  n140 = Number To Fractional String(number=w52, precision (6)=w49) -> (F-format string=w50:string)  [unwired: 2 in]
  n141 = Equal?(x=w62, y="VIVO" ("Measurement Type")) -> (x = y?=w103:bool)
  n142 = Equal?(x=w62, y="VITRO" ("Measurement Type")) -> (x = y?=w99:bool)
  n143 = Number To Fractional String(number=w25, precision (6)=w8) -> (F-format string=w24:string)  [unwired: 2 in]
  n144 = Number To Fractional String(number=w31, precision (6)=w8) -> (F-format string=w30:string)  [unwired: 2 in]
  n145 = Number To Fractional String(number=w21, precision (6)=w8) -> (F-format string=w19:string)  [unwired: 2 in]
  n146 = Number To Fractional String(number=w9, precision (6)=w8) -> (F-format string=w7:string)  [unwired: 2 in]
  n147 = Number To Fractional String(number=w28, precision (6)=w8) -> (F-format string=w27:string)  [unwired: 2 in]
  n148 = Number To Fractional String(number=w85, precision (6)=w8) -> (F-format string=w113:string)  [unwired: 2 in]
  n149 = Number To Fractional String(number=w84, precision (6)=w8) -> (F-format string=w111:string)  [unwired: 2 in]
  n150 = Number To Fractional String(number=w83, precision (6)=w8) -> (F-format string=w109:string)  [unwired: 2 in]
  n151 = Number To Fractional String(number=w82, precision (6)=w8) -> (F-format string=w120:string)  [unwired: 2 in]
  n152 = Number To Fractional String(number=w81, precision (6)=w108) -> (F-format string=w122:string)  [unwired: 2 in]
  n153 = Number To Fractional String(number=w80, precision (6)=w8) -> (F-format string=w125:string)  [unwired: 2 in]
  n154 = Number To Fractional String(number=1024.0, precision (6)=w108) -> (F-format string=w127:string)  [unwired: 2 in]
  n155 = Number To Fractional String(number=w78, precision (6)=w8) -> (F-format string=w129:string)  [unwired: 2 in]
  n156 = Number To Fractional String(number=w77, precision (6)=i16 4) -> (F-format string=w132:string)  [unwired: 2 in]
  n157 = Number To Fractional String(number=w76, precision (6)=i16 6) -> (F-format string=w134:string)  [unwired: 2 in]
  n158 = Number To Fractional String(number=w75, precision (6)=w8) -> (F-format string=w136:string)  [unwired: 2 in]
  n159 = Number To Fractional String(number=w73, precision (6)=w33) -> (F-format string=w159:string)  [unwired: 2 in]
  n160 = Number To Fractional String(number=w72, precision (6)=w33) -> (F-format string=w157:string)  [unwired: 2 in]
  n161 = Number To Fractional String(number=w71, precision (6)=w33) -> (F-format string=w155:string)  [unwired: 2 in]
  n162 = Number To Fractional String(number=w70, precision (6)=w33) -> (F-format string=w153:string)  [unwired: 2 in]
  n163 = Number To Fractional String(number=w69, precision (6)=w33) -> (F-format string=w162:string)  [unwired: 2 in]
  n164 = Select(t=w95, s=w99, f="") -> (s? t:f=w94:string)
  n165 = Concatenate Strings(w61, w100, w60, w100, w59) -> (w101:string)
  n166 = Concatenate Strings(w41, w64) -> (w90:string)
  n167 = Select(t=w101, s=w103, f=w58) -> (s? t:f=w98:string)
  n168 = Path To String(path=w44) -> (string=w47:string)
  n169 = Concatenate Strings(w47, "\\BAD_SCANS" ("string")) -> (w45:string)
  n170 = String To Path(string=w45) -> (path=w42:path)
  n171 = Search and Replace String(replace all?=TRUE ("replace all? (F)"), input string=w88, search string="\n", replace string="<CR>" ("replace string (\"\")")) -> (result string=w117:string)  [unwired: 1 in, 6 out]
  n172 = Select(t=w42, s=w37, f=w44) -> (s? t:f=w43:path)
  n173 = Transpose Matrix(1:w66) -> (0:w67:dbl[][])
  n174 = call "Format 2D Array into CharX-Separated Lines.vi"("2D Matrix"=w67, "delimiter (Tab)"="," ("data delimiter (Tab)")) -> ("String"=w139:string)
  n175 = call "Get and Format Time (String).vi"() -> ("Formatted Time"=w48:string)
  n176 = Concatenate Strings(w91, w48, w3, "Comments: " ("string"), w117, w3, "Collected with " ("string"), w17, w3, "Hardware ID: " ("string"), w15, w3, "Scripting Filename: " ("string"), w13, w3, "Magnet Type: " ("string"), w1, w3, "DAQ Mode: " ("string"), w11, w3, "Mode In-phase,Out-of-phase" ("string"), w3, "Sensitivity " ("string"), w86, w3, "Reference phase/deg " ("string"), w113, w3, "Magnetic field modulation amplitude/Gauss " ("string"), w111, w3, "Modulation Gauss /Vrms calibrated " ("string"), w109, w3, "Magnetic field modulation frequency/Hertz " ("string"), w120, w3, "Attenuation/dB " ("string"), w122, w3, "Time constant " ("string"), w87, w3, "Scan time/seconds " ("string"), w125, w3, "No. samples/scan " ("string"), w127, w3, "Scan range/Gauss " ("string"), w129, w3, "Conversion factor Gauss/V DAQ card " ("string"), w132, w3, "RF frequency/GHz " ("string"), w134, w3, "Electromagnet Main Field [G] " ("string"), w7, w3, "Central field/Gauss " ("string"), w136, w3, "Balance Scaling Factor: " ("string"), w30, w3, "Phase Error Scaling Factor: " ("string"), w27, w3, "AFC Error Scaling Factor: " ("string"), w24, w3, "AFC Field Conversion [V/MHz]: " ("string"), w19, w3, "Freq Voltage: " ("string"), w159, w3, "Phase Voltage: " ("string"), w157, w3, "In Phase Offset: " ("string"), w155, w3, "Out Phase Offset: " ("string"), w153, w3, "Q Start: " ("string"), w162, w107, w65, "***\r\n" ("string"), w139) -> (w138:string)
  n177 = Path to Array of Strings(0:w43) -> (2:w142:string[])  [unwired: 1 out]
  n178 = Concatenate Strings(w90, w104, w63, w105, w62, w105, w98, w105, w57, w105, w94, w105, w54, w104, w51, w104, w50, w105) -> (w141:string)
  n179 = Array Size(array=w142) -> (size(s)=w89:i32)
  n180 = Format Into String(format string="%s%s", initial string=w141, w48, ".ask" ("input 2")) -> (resulting string=w147:string)  [unwired: 1 in, 1 out]
  "Filename" <- w147
  n181 = Insert Into Array(array=w142, index=w89, new element=w147) -> (w148:string[])
  n182 = Array of Strings to Path(0:w148, 1:FALSE ("relative")) -> (2:w149:path)
  n183 = case shown="False" w35 {
    tunnel: w149 -> [w385 _]
    tunnel: w138 -> [w384 _]
    frame False {
      n184 = call <vilib>:"Write Characters To File.vi"("append to file? (new file:F)"=TRUE, "character string"=w384, "file path (dialog if empty)"=w385) -> ()  [unwired: 3 out]
    }
    frame True {
    }
  }
